vi "Do.vi"(8 "error in":errorcluster, 10 "Actor in":refnum<class "Actor.lvclass">, 11 "Deactivate DER Msg":refnum<class "Deactivate DER Msg.lvclass">) -> (0 "error out":errorcluster, 2 "Actor out":refnum<class "Actor.lvclass">)   [LabVIEW 2018, in "DER Actor.lvlib" / "Deactivate DER Msg.lvclass"]
doc: "(<B>Filename</B>: Actor Framework.lvlib:Message.lvclass:Do.vi)\n\nDefines what a message does when it is received by an actor. Generally, a message instructs an actor to invoke one of its methods. By default, this method does nothing. A child class must override it to define behavior. Create a child class by using the Actor Framework Message Maker dialog box."
uses:
  Deactivate DER Msg.lvclass
  <vilib>/ActorFramework/Actor/Actor.lvclass
  DER/DER.lvclass
  C:/Program Files (x86)/National Instruments/LabVIEW 2018/vi.lib/ActorFramework/Actor/Actor.lvclass
  C:/Users/Administrator/Desktop/2018LabVIEW EMS/IED Actors/Device DDS Communications Framework/Device DDS Communications/Device DDS Communications.lvclass
  Deactivate DER Msg.lvclass/Deactivate DER Msg.ctl
  <vilib>/ORNL/CSEISMIC DDS/CSEISMIC DDS Base/Data Types/DER_Control.ctl
  <vilib>/ORNL/CSEISMIC DDS/CSEISMIC DDS Base/Data Types/Controls/DeviceID.ctl
  Device DDS Communications Framework/Device DDS Communications/Device DDS Communications.lvclass/Device DDS Communications.ctl
  <vilib>/ORNL/CSEISMIC DDS/CSEISMIC DDS Base/CSEISMIC DDS.lvclass/CSEISMIC DDS.ctl
  <vilib>/ORNL/CSEISMIC DDS/DDS Writer/Writers/Write DER_Control.vi
  Device DDS Communications Framework/Device DDS Communications/Accessors/Read DDS Writer Object.vi
  <vilib>/ORNL/CSEISMIC DDS/CSEISMIC DDS Base/Accessors/Read DDS Reference.vi
  <vilib>/ORNL/CSEISMIC DDS/DDS Writer/DDS Writer.lvclass
  C:/Program Files (x86)/National Instruments/LabVIEW 2018/vi.lib/ORNL/CSEISMIC DDS/CSEISMIC DDS Base/CSEISMIC DDS.lvclass
  <vilib>/ORNL/CSEISMIC DDS/CSEISMIC DDS Base/Error Handler.vi
  <vilib>/ORNL/CSEISMIC DDS/CSEISMIC DDS Base/CSEISMIC DDS.lvclass
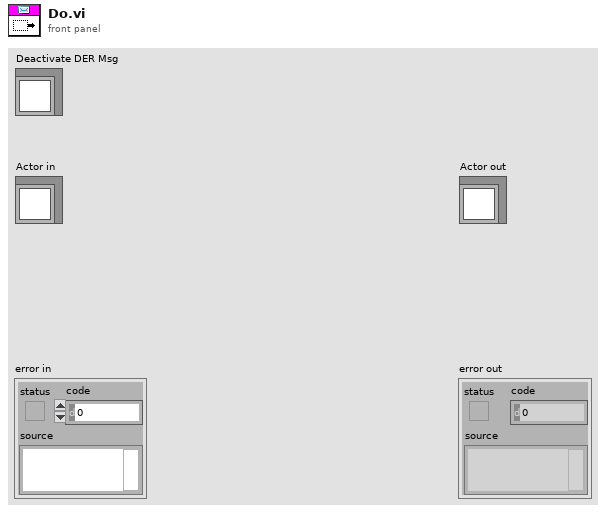
[diagram p1: front panel]
types:
  T1 = typedef "CSEISMIC DDS.lvlib/CSEISMIC DDS.lvclass/DeviceID.ctl" = string
  T2 = typedef "CSEISMIC DDS.lvlib/CSEISMIC DDS.lvclass/DER_Control.ctl" = cluster{"DeviceID":T1, "Activate":bool, "Deactivate":bool}
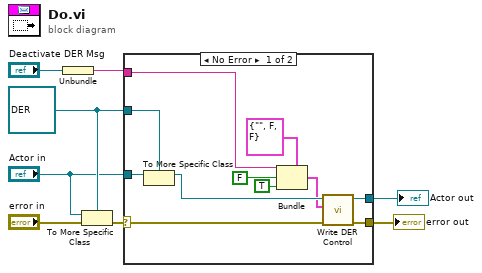
[diagram p0: block diagram]
diagram:
  w8 = refnum<class "DER.lvclass"> refnum ("DER Actor.lvlib:DER.lvclass")
  n1 = Unbundle("Deactivate DER Msg") -> (w1:T1)
  n2 = To More Specific Class(target class=w8, reference="Actor in", error in="error in") -> (error out=w6:errorcluster)  [unwired: 1 out]
  n3 = case shown="No Error" w6 {
    selector: w6 -> [w17 w21]
    tunnel: [w19 w21] -> w4
    tunnel: [w18 w20] -> w3
    tunnel: "Actor in" -> [w16 w20]
    tunnel: w8 -> [w15 _]
    tunnel: w1 -> [w11 _]
    frame No Error {
      n4 = To More Specific Class(target class=w15, reference=w16) -> (specific class reference=w14:refnum<class "DER.lvclass">)  [unwired: 1 in, 1 out]
      n5 = Bundle(cluster=T2 {"DeviceID"="", "Activate"=FALSE, "Deactivate"=FALSE} ("DER_Control"), "DeviceID"=w11, "Activate"=FALSE, "Deactivate"=TRUE) -> (w12:T2)
      n6 = call "Write DER Control.vi"("error in"=w17, "DER_Control"=w12, "DER in"=w14) -> ("error out"=w19:errorcluster, "DER out"=w18:refnum<class "DER.lvclass">)  [unwired: 7 in]
    }
    frame Error {
      # "If type check fails, pass the original object out again."
    }
  }
  "error out" <- w4
  "Actor out" <- w3
